vi "Initialize Control.vi"(8 "error in (no error)":errorcluster, 11 "ColorSelector in":refnum<class "ColorSelector.lvclass">) -> (0 "error out":errorcluster, 3 "ColorSelector out":refnum<class "ColorSelector.lvclass">)   [LabVIEW 2020, in "ColorSelector.lvclass"]
doc: "The <b>Initialize VI</b> is a dynamic dispatch VI that must be overwritten in every QControl Class. It must <b>Call Parent Method</b> so that it recursively calls the initialize routine all of the way up the inheritance hierarchy. \n\nThe top most call is to the <b>Initialize Control VI</b> in Control.lvclass. This is the VI that starts the <b>Event Handler VI</b> if there was one overwritten in the QControl.\n<b> </b> <b> </b>\n©2017 Q Software Innovations, LLC (QSI)\nwritten by Quentin Alldredge\nproduced in LabVIEW 2015\n\nsupport@qsoftwareinnovations.com\nwww.qsoftwareinnovations.com\n\nAll rights reserved.\n\nRedistribution and use in source and binary forms, with or without modification, are permitted provided that the following conditions are met:\n\n * Redistributions of source code must retain the above copyright notice, this list of conditions and the following disclaimer.\n * Redistributions in binary form must reproduce the above copyright notice, this list of conditions and the following disclaimer in the documentation and/or other materials provided with the distribution.\n * Neither the name of Q Software Innovations, LLC. nor the names of its contributors may be used to endorse or promote products derived from this software without specific prior written permission.\n\nTHIS SOFTWARE IS PROVIDED BY THE COPYRIGHT HOLDERS AND CONTRIBUTORS \"AS IS\" AND ANY EXPRESS OR IMPLIED WARRANTIES, INCLUDING, BUT NOT LIMITED TO, THE IMPLIED WARRANTIES OF MERCHANTABILITY AND FITNESS FOR A PARTICULAR PURPOSE ARE DISCLAIMED. IN NO EVENT SHALL THE COPYRIGHT OWNER OR CONTRIBUTORS BE LIABLE FOR ANY DIRECT, INDIRECT, INCIDENTAL, SPECIAL, EXEMPLARY, OR CONSEQUENTIAL DAMAGES (INCLUDING, BUT NOT LIMITED TO, PROCUREMENT OF SUBSTITUTE GOODS OR SERVICES; LOSS OF USE, DATA, OR PROFITS; OR BUSINESS INTERRUPTION) HOWEVER CAUSED AND ON ANY THEORY OF LIABILITY, WHETHER IN CONTRACT, STRICT LIABILITY, OR TORT (INCLUDING NEGLIGENCE OR OTHERWISE) ARISING IN ANY WAY OUT OF THE USE OF THIS SOFTWARE, EVEN IF ADVISED OF THE POSSIBILITY OF SUCH DAMAGE."
uses:
  ColorSelector.lvclass
  <vilib>/Utility/miscctls.llb/LVPoint32TypeDef.ctl
  ColorSelector.lvclass/ColorSelector.ctl
  <vilib>/QSI/QControls/QControl Classes/Cluster/Cluster.lvclass
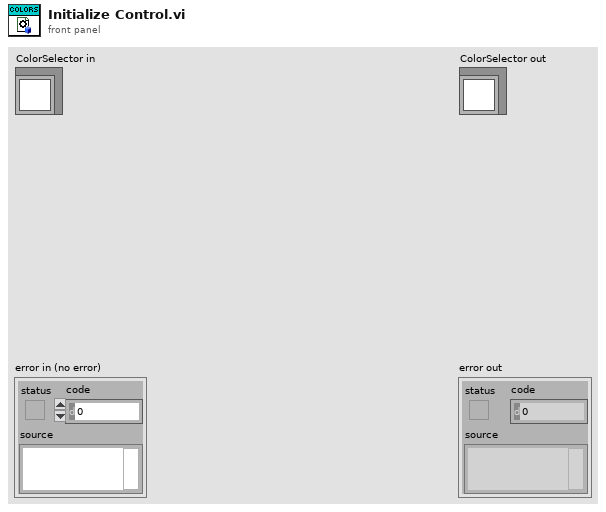
[diagram p1: front panel]
types:
  T1 = typedef "LVPoint32TypeDef.ctl" = cluster{"Horizontal":i32, "Vertical":i32}
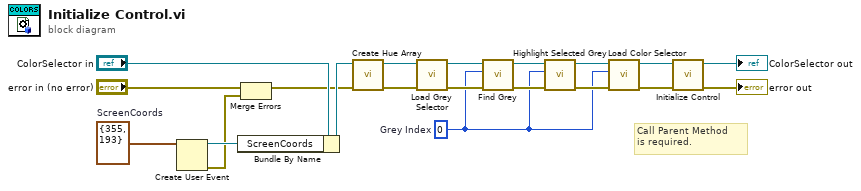
[diagram p0: block diagram]
diagram:
  w13 = T1 {"Horizontal"=355, "Vertical"=193}  # ScreenCoords
  w1 = u8 0  # Grey Index
  # "Call Parent Method\nis required."
  n1 = Create User Event(user event datatype=w13) -> (user event=w12:refnum<user-event>, error out=w8:errorcluster)  [unwired: 1 in]
  n2 = Bundle By Name(cluster="ColorSelector in", "ScreenCoords"=w12) -> (w10:refnum<class "ColorSelector.lvclass">)
  n3 = Merge Errors("error in (no error)", w8) -> (w9:errorcluster)
  n4 = call "Create Hue Array.vi"("error in (no error)"=w9, "ColorSelector in"=w10) -> ("error out"=w16:errorcluster, "ColorSelector out"=w18:refnum<class "ColorSelector.lvclass">)  [unwired: 8 in]
  n5 = call "Load Grey Selector.vi"("error in (no error)"=w16, "ColorSelector in"=w18) -> ("error out"=w3:errorcluster, "ColorSelector out"=w5:refnum<class "ColorSelector.lvclass">)  [unwired: 8 in]
  n6 = call "Find Grey.vi"("error in (no error)"=w3, "Grey Index (0-255)"=w1, "ColorSelector in"=w5) -> ("error out"=w2:errorcluster, "ColorSelector out"=w4:refnum<class "ColorSelector.lvclass">)  [unwired: 7 in]
  n7 = call "Highlight Selected Grey.vi"("error in (no error)"=w2, "Grey Scale Index (0-255)"=w1, "ColorSelector in"=w4) -> ("error out"=w6:errorcluster, "ColorSelector (dup)"=w7:refnum<class "ColorSelector.lvclass">)  [unwired: 7 in]
  n8 = call "Load Color Selector.vi"("error in (no error)"=w6, "Grey Scale Index (0-255)"=w1, "ColorSelector in"=w7) -> ("error out"=w14:errorcluster, "ColorSelector out"=w15:refnum<class "ColorSelector.lvclass">)  [unwired: 7 in]
  n9 = call-parent "Initialize Control.vi"("error in (no error)"=w14, "Control in"=w15) -> ("error out"=→"error out":errorcluster, "Control out"=→"ColorSelector out":refnum<class "ColorSelector.lvclass">)  [unwired: 8 in]
